vi "Module Did Stop.vi"(8 "error in":errorcluster, 10 "Origin":string, 11 "Module ID":i32=-1) -> (0 "error out":errorcluster)   [LabVIEW 2022 SP3, in "HW-210_dqmh.lvlib"]
doc: "Send the Module Did Stop event to any VI registered to listen to this module's broadcast events.\n_____\nBased on DQMH Project Template 7.0.1.1316."
uses:
  HW-210_dqmh.lvlib
  Stop Argument--cluster.ctl
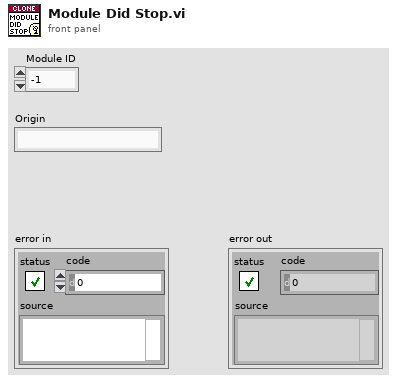
[diagram p1: front panel]
types:
  T1 = typedef "HW-210_dqmh.lvlib/Stop Argument--cluster.ctl" = cluster{"Module ID":i32, "Origin":string, "Exit via Stop Module Req?":bool, "Wait for Module to stop?":bool}
  T2 = typedef "HW-210_dqmh.lvlib/Broadcast Events--cluster.ctl" = cluster{"Module Did Init":refnum<user-event>, "Status Updated":refnum<user-event>, "Error Reported":refnum<user-event>, "Module Did Stop":refnum<user-event>, "Update Module Execution Status":refnum<user-event>, "Linx":refnum<user-event>}
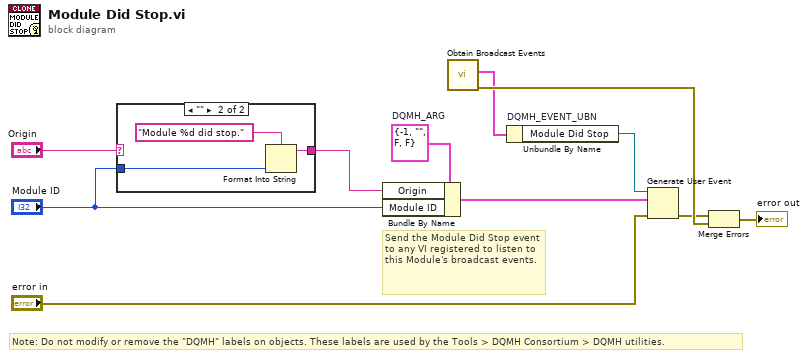
[diagram p0: block diagram]
diagram:
  w4 = T1 {"Module ID"=-1, "Origin"="", "Exit via Stop Module Req?"=FALSE, "Wait for Module to stop?"=FALSE}  # DQMH_ARG
  # "Note: Do not modify or remove the \"DQMH\" labels on objects. These labels are used by the Tools > DQMH Consortium > DQMH utilities."
  # "Send the Module Did Stop event to any VI registered to listen to this Module's broadcast events."
  n1 = case shown="\"\"" "Origin" {
    selector: "Origin" -> [w12 _]
    tunnel: "Module ID" -> [_ w15]
    tunnel: [w12 w13] -> w2
    frame Default {
    }
    frame "" {
      n2 = Format Into String(format string="Module %d did stop.", w15) -> (resulting string=w13:string)  [unwired: 2 in, 1 out]
    }
  }
  n3 = Bundle By Name(cluster=w4, "Origin"=w2, "Module ID"="Module ID") -> (w5:T1)
  n4 = call "Obtain Broadcast Events.vi"() -> ("error out"=w9:errorcluster, "HW-210 Broadcast Events"=w7:T2)  [unwired: 10 in]
  n5 = Unbundle By Name "DQMH_EVENT_UBN"(w7) -> ("Module Did Stop"=w6:refnum<user-event>)
  n6 = Generate User Event(user event=w6, event data cluster=w5, error in="error in") -> (error out=w8:errorcluster)  [unwired: 1 in, 1 out]
  n7 = Merge Errors(w8, w9) -> (→"error out":errorcluster)
